vi "logicaSecuencial.vi"() -> ()   [LabVIEW 2010]
uses:
  <vilib>/Analysis/NI_AALBase.lvlib
  CaseControl.ctl
panel:
  in  "Señal Actual":dbl[](array[numeric])
  in  "Parametros Control":T1
  in  "Parametros Iniciales":T2
  out "ControlCase OUT":T3 items=["00 - Promedio Inicial", "01 - Genera señal aleatoria", "02 - Incrementa t0", "03 - Promedia buen t0", "04 - Inicializa Amplitud", "05 - Incrementa Amplitud", "06 - Promedia buena Amplitud", "07 - Inicializa Sigma", "08 - Incrementa Sigma", "09 - Promedia buen Sigma", "10 - Actualiza mejor señal", "11 - Control ON, Ajuste OFF", "12 - Control OFF"]
  in  "ControlCase IN":T3 items=["00 - Promedio Inicial", "01 - Genera señal aleatoria", "02 - Incrementa t0", "03 - Promedia buen t0", "04 - Inicializa Amplitud", "05 - Incrementa Amplitud", "06 - Promedia buena Amplitud", "07 - Inicializa Sigma", "08 - Incrementa Sigma", "09 - Promedia buen Sigma", "10 - Actualiza mejor señal", "11 - Control ON, Ajuste OFF", "12 - Control OFF"]
  in  "Contraste":dbl
  out "Señal de Control OUT":dbl[](array[numeric])
  in  "Señal de Control IN":dbl[](array[numeric])
  in  "Parametros Actuales":T2
  out "Mejores Parametros OUT":T2
  in  "Mejores Parametros IN":T2
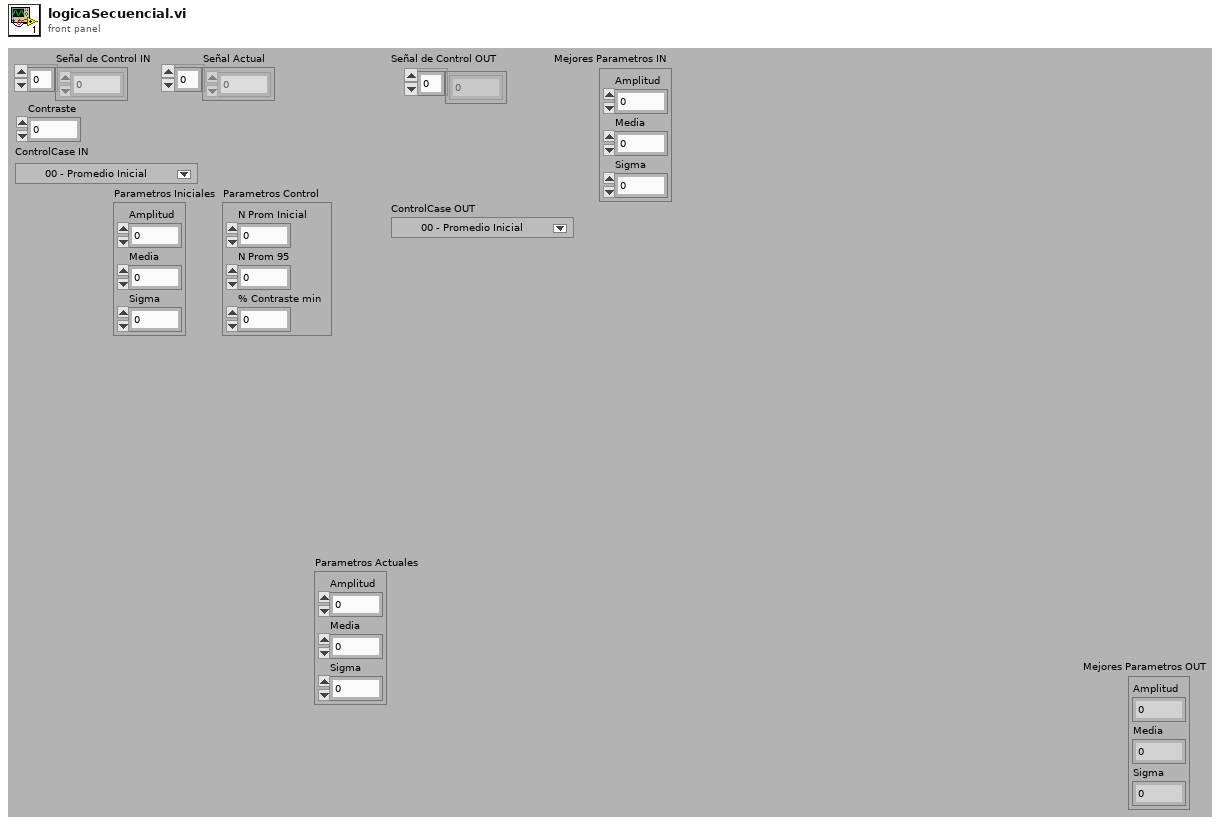
[diagram p1: front panel]
types:
  T1 = cluster{"N Prom Inicial":u32, "N Prom 95":u32, "% Contraste min":dbl}
  T2 = cluster{"Amplitud":dbl, "Media":dbl, "Sigma":dbl}
  T3 = typedef "CaseControl.ctl" = u32
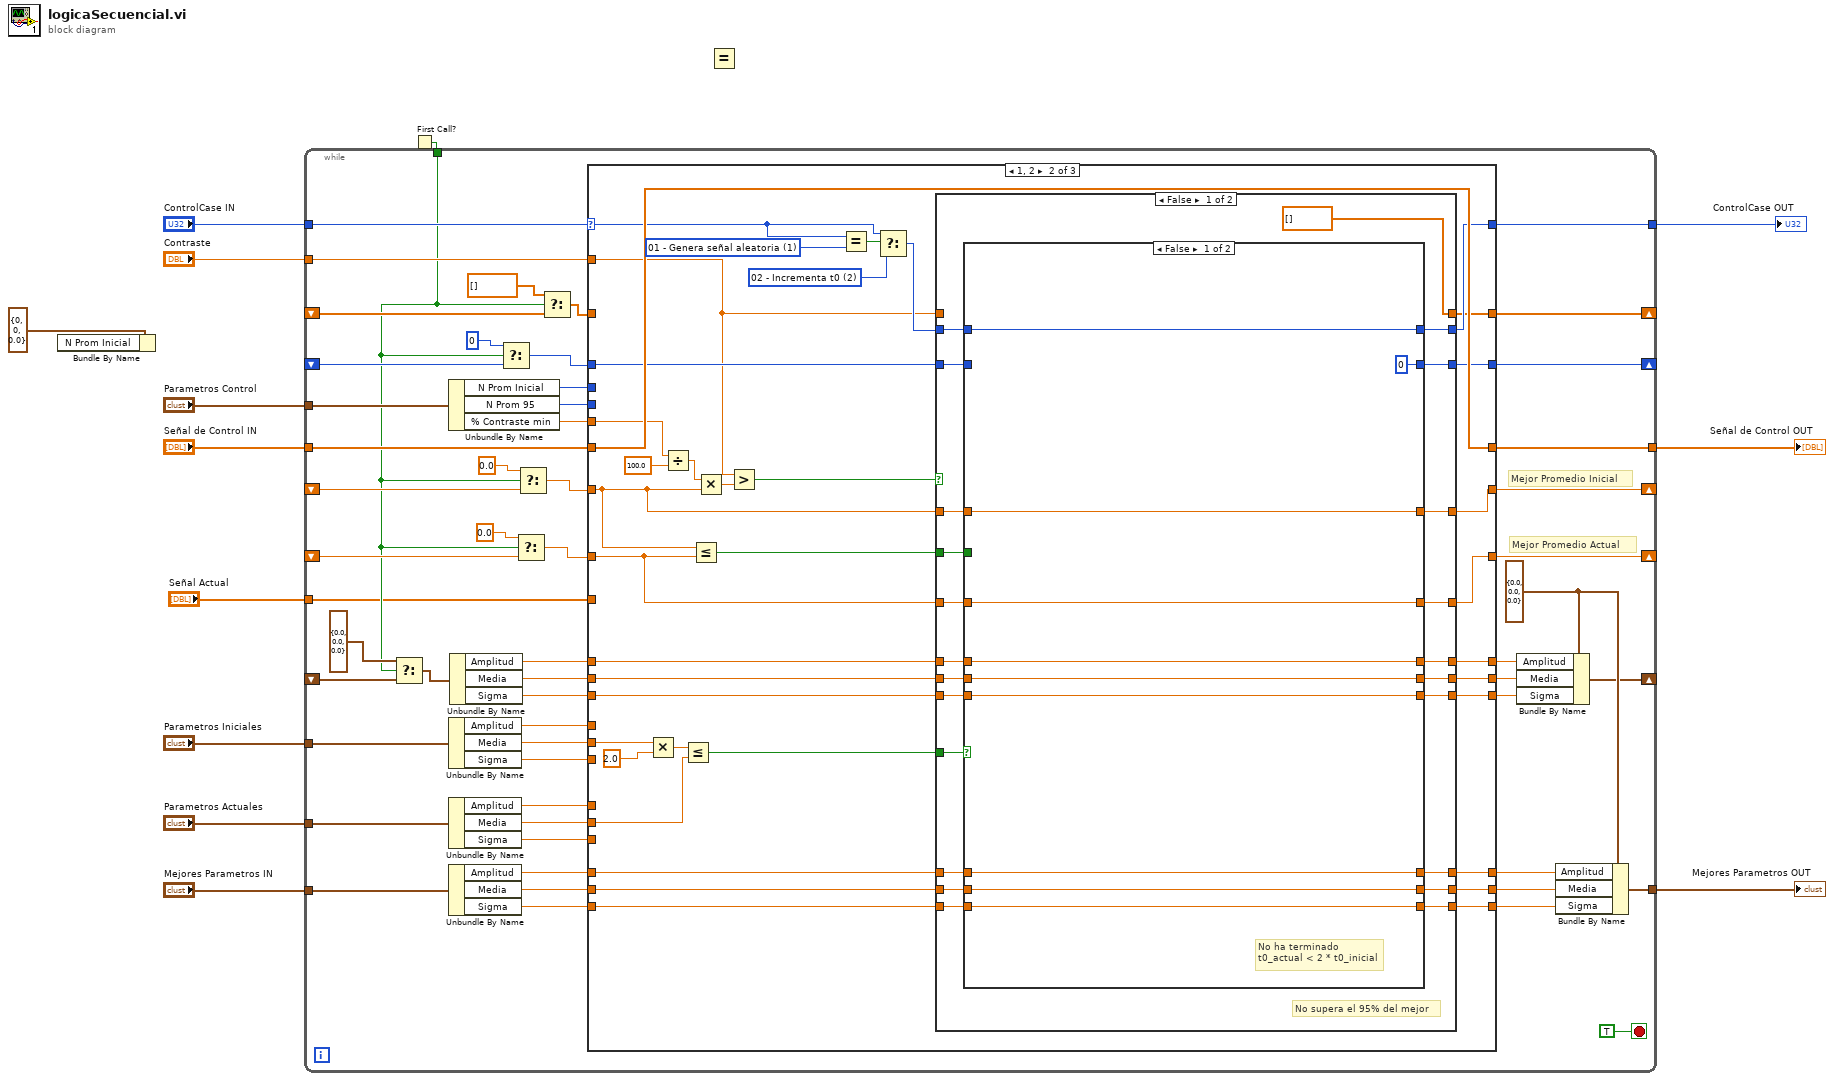
[diagram p0: block diagram]
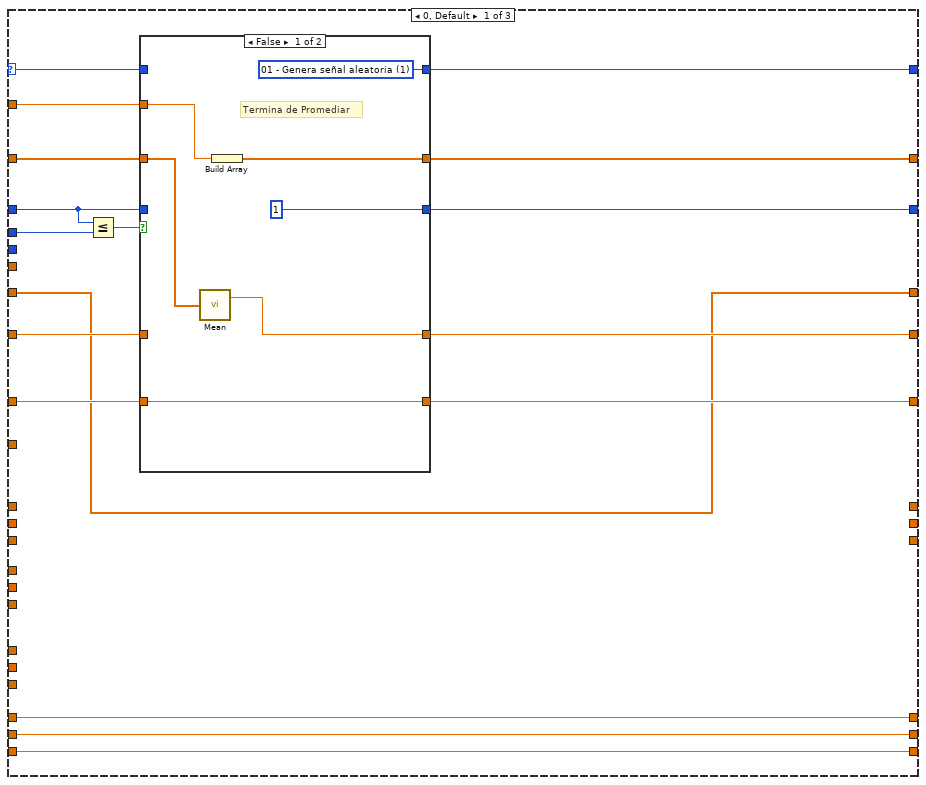
[diagram p2: hidden frame]
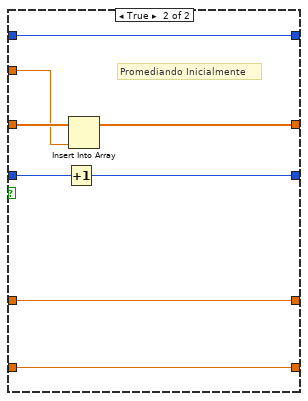
[diagram p3: hidden frame]
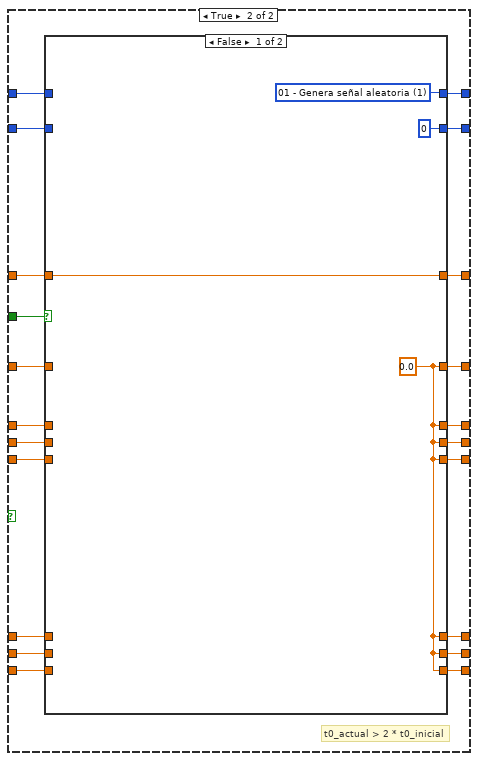
[diagram p4: hidden frame]
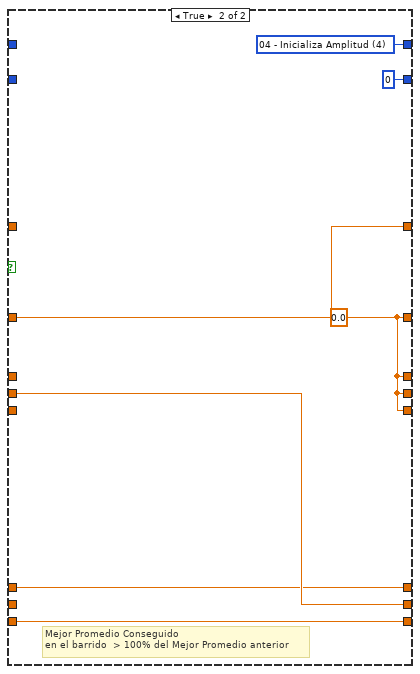
[diagram p5: hidden frame]
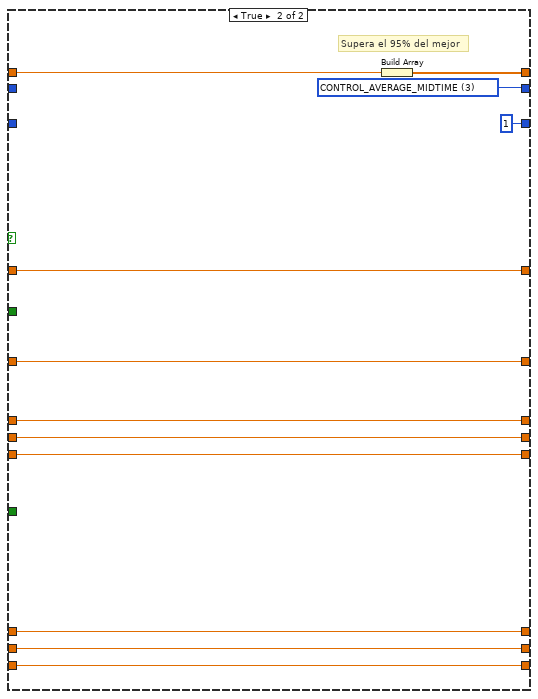
[diagram p6: hidden frame]
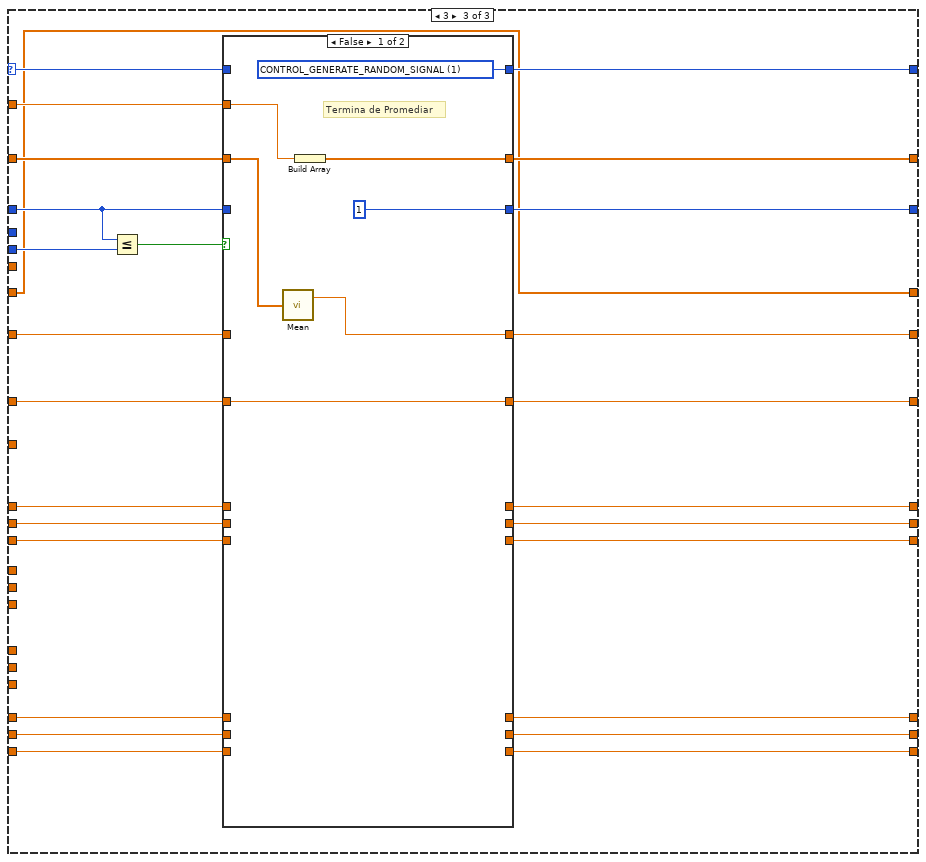
[diagram p7: hidden frame]
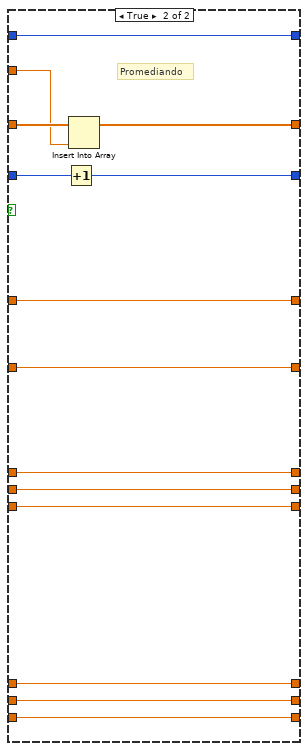
[diagram p8: hidden frame]
diagram:
  n1 = Bundle By Name(cluster=T1 {"N Prom Inicial"=0, "N Prom 95"=0, "% Contraste min"=0.0} ("input cluster")) -> ()  [unwired: 1 in, 1 out]
  n2 = First Call?() -> (First Call?: T/F=w6:bool)
  n3 = while {
    tunnel: "Mejores Parametros IN" -> [w68]
    tunnel: [w67] -> w12
    tunnel: "Parametros Actuales" -> [w66]
    tunnel: "Señal de Control IN" -> [w63]
    tunnel: [w62] -> w9
    tunnel: "Contraste" -> [w46]
    tunnel: "ControlCase IN" -> [w64]
    tunnel: w6 -> [w20]
    shift-right: [w50] -> _
    shift-left: _ -> [w49]
    shift-right: [w42] -> _
    shift-left: _ -> [w44]
    tunnel: [w41] -> w4
    shift-right: [w40] -> _
    shift-left: _ -> [w38]
    shift-right: [w34] -> _
    shift-left: _ -> [w35]
    tunnel: "Parametros Iniciales" -> [w32]
    tunnel: "Parametros Control" -> [w28]
    shift-right: [w25] -> _
    shift-left: _ -> [w19]
    tunnel: "Señal Actual" -> [w14]
    stop <- TRUE stop-if-true
    w26 = T2 {"Amplitud"=0.0, "Media"=0.0, "Sigma"=0.0} ("input cluster")
    # "Mejor Promedio Inicial"
    # "Mejor Promedio Actual"
    n4 = Select(t=T2 {"Amplitud"=0.0, "Media"=0.0, "Sigma"=0.0} ("input cluster"), s=w20, f=w19) -> (s? t:f=w18:T2)
    n5 = Unbundle By Name(w28) -> ("N Prom Inicial"=w48:u32, "N Prom 95"=w47:u32, "% Contraste min"=w27:dbl)
    n6 = Unbundle By Name(w32) -> ("Amplitud"=w31:dbl, "Media"=w30:dbl, "Sigma"=w29:dbl)
    n7 = Unbundle By Name(w66) -> ("Amplitud"=w61:dbl, "Media"=w60:dbl, "Sigma"=w59:dbl)
    n8 = Unbundle By Name(w68) -> ("Amplitud"=w58:dbl, "Media"=w55:dbl, "Sigma"=w53:dbl)
    n9 = Unbundle By Name(w18) -> ("Amplitud"=w24:dbl, "Media"=w23:dbl, "Sigma"=w22:dbl)
    n10 = Select(t=0, s=w20, f=w49) -> (s? t:f=w51:i32)
    n11 = Select(t=0.0, s=w20, f=w35) -> (s? t:f=w33:dbl)
    n12 = Select(t=0.0, s=w20, f=w38) -> (s? t:f=w37:dbl)
    n13 = Select(t=dbl[] [], s=w20, f=w44) -> (s? t:f=w43:dbl[])
    n14 = case shown="1, 2" w64 {
      selector: w64 -> [w78 w127 w236]
      tunnel: w63 -> [w69 w138 w232]
      tunnel: [w69 w138 w232] -> w62
      tunnel: w61 -> [_ _ _]
      tunnel: w60 -> [_ w129 _]
      tunnel: w59 -> [_ _ _]
      tunnel: w58 -> [w72 w111 w220]
      tunnel: [w72 w112 w221] -> w57
      tunnel: [w71 w110 w219] -> w56
      tunnel: w55 -> [w71 w109 w218]
      tunnel: [w70 w108 w217] -> w54
      tunnel: w53 -> [w70 w107 w216]
      tunnel: w51 -> [w83 w105 w239]
      tunnel: [w82 w106 w233] -> w50
      tunnel: w48 -> [w85 _ _]
      tunnel: w47 -> [_ _ w241]
      tunnel: w46 -> [w79 w103 w238]
      tunnel: w43 -> [w81 _ w237]
      tunnel: [w80 w104 w234] -> w42
      tunnel: [w77 w123 w235] -> w41
      tunnel: [w76 w120 w229] -> w40
      tunnel: w37 -> [w75 w119 w231]
      tunnel: [w74 w122 w228] -> w34
      tunnel: w33 -> [w73 w121 w230]
      tunnel: w31 -> [_ _ _]
      tunnel: w30 -> [_ w130 _]
      tunnel: w29 -> [_ _ _]
      tunnel: w27 -> [_ w134 _]
      tunnel: w24 -> [_ w118 w226]
      tunnel: w23 -> [_ w117 w224]
      tunnel: w22 -> [_ w116 w222]
      tunnel: [_ w115 w227] -> w17
      tunnel: [_ w114 w225] -> w16
      tunnel: [_ w113 w223] -> w15
      tunnel: w14 -> [_ _ _]
      frame 0, Default {
        n15 = Less Or Equal?(x=w83, y=w85) -> (x <= y?=w84:bool)
        n16 = case shown="False" w84 {
          tunnel: w83 -> [_ w100]
          tunnel: [1 w99] -> w82
          tunnel: [w91 w97] -> w80
          tunnel: w81 -> [w89 w98]
          tunnel: w79 -> [w90 w96]
          tunnel: w78 -> [_ w95]
          tunnel: [w86 w95] -> w77
          tunnel: [w88 w94] -> w76
          tunnel: w75 -> [_ w94]
          tunnel: [w87 w93] -> w74
          tunnel: w73 -> [w87 w93]
          frame False {
            w86 = T3 1 items=["00 - Promedio Inicial", "01 - Genera señal aleatoria", "02 - Incrementa t0", "03 - Promedia buen t0", "04 - Inicializa Amplitud", "05 - Incrementa Amplitud", "06 - Promedia buena Amplitud", "07 - Inicializa Sigma", "08 - Incrementa Sigma", "09 - Promedia buen Sigma", "10 - Actualiza mejor señal", "11 - Control ON, Ajuste OFF", "12 - Control OFF"] ("ControlCase IN")
            # "Termina de Promediar"
            n17 = call <vilib>:"Mean.vi"("X"=w89) -> ("mean"=w88:dbl)  [unwired: 1 out]
            n18 = Build Array(w90) -> (w91:dbl[])
          }
          frame True {
            # "Promediando Inicialmente"
            n19 = Increment(x=w100) -> (x+1=w99:i32)
            n20 = Insert Into Array(array=w98, new element=w96) -> (w97:dbl[])  [unwired: 1 in]
          }
        }
      }
      frame 1, 2 {
        w101 = T3 2 items=["00 - Promedio Inicial", "01 - Genera señal aleatoria", "02 - Incrementa t0", "03 - Promedia buen t0", "04 - Inicializa Amplitud", "05 - Incrementa Amplitud", "06 - Promedia buena Amplitud", "07 - Inicializa Sigma", "08 - Incrementa Sigma", "09 - Promedia buen Sigma", "10 - Actualiza mejor señal", "11 - Control ON, Ajuste OFF", "12 - Control OFF"] ("f")
        w102 = T3 1 items=["00 - Promedio Inicial", "01 - Genera señal aleatoria", "02 - Incrementa t0", "03 - Promedia buen t0", "04 - Inicializa Amplitud", "05 - Incrementa Amplitud", "06 - Promedia buena Amplitud", "07 - Inicializa Sigma", "08 - Incrementa Sigma", "09 - Promedia buen Sigma", "10 - Actualiza mejor señal", "11 - Control ON, Ajuste OFF", "12 - Control OFF"] ("y")
        n21 = Multiply(x=w130, y=2.0 ("x")) -> (x*y=w131:dbl)
        n22 = Divide(x=w134, y=100.0) -> (x/y=w135:dbl)
        n23 = Less Or Equal?(x=w131, y=w129) -> (x <= y?=w125:bool)
        n24 = Less Or Equal?(x=w119, y=w121) -> (x <= y?=w126:bool)
        n25 = Multiply(x=w135, y=w119) -> (x*y=w133:dbl)
        n26 = Greater?(x=w103, y=w133) -> (0:w137:bool)
        n27 = Equal?(x=w127, y=w102) -> (x = y?=w128:bool)
        n28 = Select(t=w127, s=w128, f=w101) -> (s? t:f=w124:T3)
        n29 = case shown="False" w137 {
          tunnel: w126 -> [w158 _]
          tunnel: w125 -> [w159 _]
          tunnel: w124 -> [w161 _]
          tunnel: [w160 w215] -> w123
          tunnel: [w157 w207] -> w122
          tunnel: w121 -> [w156 w207]
          tunnel: [w155 w208] -> w120
          tunnel: w119 -> [w154 w208]
          tunnel: w118 -> [w153 w214]
          tunnel: w117 -> [w152 w213]
          tunnel: w116 -> [w151 w212]
          tunnel: [w150 w214] -> w115
          tunnel: [w149 w213] -> w114
          tunnel: [w148 w212] -> w113
          tunnel: [w147 w211] -> w112
          tunnel: w111 -> [w146 w211]
          tunnel: [w145 w210] -> w110
          tunnel: w109 -> [w144 w210]
          tunnel: [w143 w209] -> w108
          tunnel: w107 -> [w142 w209]
          tunnel: [w141 1] -> w106
          tunnel: w105 -> [w140 _]
          tunnel: [dbl[] [] w205] -> w104
          tunnel: w103 -> [_ w204]
          frame False {
            # "No supera el 95% del mejor"
            n30 = case shown="False" w159 {
              tunnel: w161 -> [w171 w192]
              tunnel: [w171 w190] -> w160
              tunnel: w158 -> [_ w191]
              tunnel: [w166 w189] -> w157
              tunnel: w156 -> [w166 w188]
              tunnel: [w170 w187] -> w155
              tunnel: w154 -> [w170 w186]
              tunnel: w153 -> [w169 w185]
              tunnel: w152 -> [w168 w184]
              tunnel: w151 -> [w167 w183]
              tunnel: [w169 w182] -> w150
              tunnel: [w168 w181] -> w149
              tunnel: [w167 w180] -> w148
              tunnel: [w165 w179] -> w147
              tunnel: w146 -> [w165 w178]
              tunnel: [w164 w177] -> w145
              tunnel: w144 -> [w164 w176]
              tunnel: [w163 w175] -> w143
              tunnel: w142 -> [w163 w174]
              tunnel: [0 w173] -> w141
              tunnel: w140 -> [_ w172]
              frame False {
                # "No ha terminado\nt0_actual < 2 * t0_inicial"
              }
              frame True {
                # "t0_actual > 2 * t0_inicial"
                n31 = case shown="False" w191 {
                  tunnel: w192 -> [_ _]
                  tunnel: [w193 w197] -> w190
                  tunnel: [w195 w200] -> w189
                  tunnel: w188 -> [_ w199]
                  tunnel: [w196 w199] -> w187
                  tunnel: w186 -> [w196 _]
                  tunnel: w185 -> [_ _]
                  tunnel: w184 -> [_ w203]
                  tunnel: w183 -> [_ _]
                  tunnel: [w195 w200] -> w182
                  tunnel: [w195 w200] -> w181
                  tunnel: [w195 w200] -> w180
                  tunnel: [w195 w202] -> w179
                  tunnel: w178 -> [_ w202]
                  tunnel: [w195 w203] -> w177
                  tunnel: w176 -> [_ _]
                  tunnel: [w195 w201] -> w175
                  tunnel: w174 -> [_ w201]
                  tunnel: [0 0] -> w173
                  tunnel: w172 -> [_ _]
                  frame False {
                    w193 = T3 1 items=["00 - Promedio Inicial", "01 - Genera señal aleatoria", "02 - Incrementa t0", "03 - Promedia buen t0", "04 - Inicializa Amplitud", "05 - Incrementa Amplitud", "06 - Promedia buena Amplitud", "07 - Inicializa Sigma", "08 - Incrementa Sigma", "09 - Promedia buen Sigma", "10 - Actualiza mejor señal", "11 - Control ON, Ajuste OFF", "12 - Control OFF"] ("f")
                    w195 = 0.0
                  }
                  frame True {
                    w197 = T3 4 items=["00 - Promedio Inicial", "01 - Genera señal aleatoria", "02 - Incrementa t0", "03 - Promedia buen t0", "04 - Inicializa Amplitud", "05 - Incrementa Amplitud", "06 - Promedia buena Amplitud", "07 - Inicializa Sigma", "08 - Incrementa Sigma", "09 - Promedia buen Sigma", "10 - Actualiza mejor señal", "11 - Control ON, Ajuste OFF", "12 - Control OFF"] ("f")
                    w200 = 0.0
                    # "Mejor Promedio Conseguido \nen el barrido  > 100% del Mejor Promedio anterior"
                  }
                }
              }
            }
          }
          frame True {
            w215 = T3 3 items=["CONTROL_INITIAL_AVERAGE", "CONTROL_GENERATE_RANDOM_SIGNAL", "CONTROL_INCREMENT_MIDTIME", "CONTROL_AVERAGE_MIDTIME", "CONTROL_INITIATE_AMPLITUDE", "CONTROL_INCREMENT_AMPLITUDE", "CONTROL_AVERAGE_AMPLITUDE", "CONTROL_INITIATE_SIGMA", "CONTROL_INCREMENT_SIGMA", "CONTROL_AVERAGE_SIGMA", "CONTROL_BEST_SIGNAL", "CONTROL_ADJUST_OFF", "CONTROL_OFF"] ("ControlCase")
            # "Supera el 95% del mejor"
            n32 = Build Array(w204) -> (w205:dbl[])
          }
        }
      }
      frame 3 {
        n33 = Less Or Equal?(x=w239, y=w241) -> (x <= y?=w240:bool)
        n34 = case shown="False" w240 {
          tunnel: w239 -> [_ w262]
          tunnel: [1 w261] -> w233
          tunnel: [w247 w259] -> w234
          tunnel: w237 -> [w245 w260]
          tunnel: w238 -> [w246 w258]
          tunnel: w236 -> [_ w257]
          tunnel: [w242 w257] -> w235
          tunnel: [w244 w256] -> w229
          tunnel: w231 -> [_ w256]
          tunnel: [w243 w255] -> w228
          tunnel: w230 -> [w243 w255]
          tunnel: [_ w254] -> w227
          tunnel: w226 -> [_ w254]
          tunnel: [_ w253] -> w225
          tunnel: w224 -> [_ w253]
          tunnel: [_ w252] -> w223
          tunnel: w222 -> [_ w252]
          tunnel: [_ w251] -> w221
          tunnel: w220 -> [_ w251]
          tunnel: [_ w250] -> w219
          tunnel: w218 -> [_ w250]
          tunnel: [_ w249] -> w217
          tunnel: w216 -> [_ w249]
          frame False {
            w242 = T3 1 items=["CONTROL_INITIAL_AVERAGE", "CONTROL_GENERATE_RANDOM_SIGNAL", "CONTROL_INCREMENT_MIDTIME", "CONTROL_AVERAGE_MIDTIME", "CONTROL_INITIATE_AMPLITUDE", "CONTROL_INCREMENT_AMPLITUDE", "CONTROL_AVERAGE_AMPLITUDE", "CONTROL_INITIATE_SIGMA", "CONTROL_INCREMENT_SIGMA", "CONTROL_AVERAGE_SIGMA", "CONTROL_BEST_SIGNAL", "CONTROL_ADJUST_OFF", "CONTROL_OFF"] ("ControlCase")
            # "Termina de Promediar"
            n35 = call <vilib>:"Mean.vi"("X"=w245) -> ("mean"=w244:dbl)  [unwired: 1 out]
            n36 = Build Array(w246) -> (w247:dbl[])
          }
          frame True {
            # "Promediando"
            n37 = Increment(x=w262) -> (x+1=w261:i32)
            n38 = Insert Into Array(array=w260, new element=w258) -> (w259:dbl[])  [unwired: 1 in]
          }
        }
      }
    }
    n39 = Bundle By Name(cluster=w26, "Amplitud"=w17, "Media"=w16, "Sigma"=w15) -> (w25:T2)
    n40 = Bundle By Name(cluster=w26, "Amplitud"=w57, "Media"=w56, "Sigma"=w54) -> (w67:T2)
  }
  "Mejores Parametros OUT" <- w12
  "Señal de Control OUT" <- w9
  "ControlCase OUT" <- w4
  n41 = Equal?() -> ()  [unwired: 2 in, 1 out]
